vi "rejectAck.vi"(8 "error in (no error)":errorcluster, 10 "InternalCommandId":refnum<class "InternalCommandId.lvclass">, 11 "ElectrometerController in":refnum<class "ElectrometerController.lvclass">) -> (0 "error out":errorcluster, 3 "ElectrometerController out":refnum<class "ElectrometerController.lvclass">)   [LabVIEW 2016, in "ElectrometerController.lvclass"]
uses:
  ElectrometerController.lvclass
  InternalCommandId/InternalCommandId.lvclass
  ts_electrometeruserevents/Typedefs/CommandValue.ctl
  ElectrometerController.lvclass/ElectrometerController.ctl
  ts_electrometeruserevents/PubSubDataEvent/PubSubDataEvent.lvclass
  ts_electrometeruserevents/Typedefs/ElectrometerTypedefs.lvlib
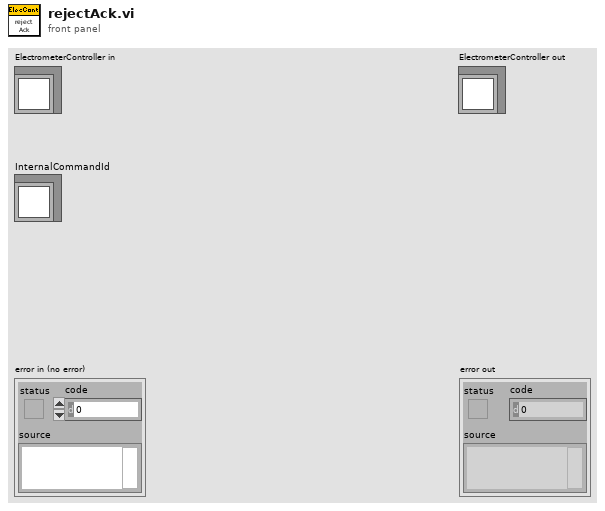
[diagram p1: front panel]
types:
  T1 = typedef "ElectrometerTypedefs.lvlib/CommandValue.ctl" = enum16{"N/A", "Disable", "Enable", "Exit", "GoToStandby", "OnHeartbeat", "OnIncomingMessagingError", "OnInterrupt", "Start", "SetDigitalFilter", "StartScan", "StartScanDt", "StartScanReachIntensity", "StopScan", "SetIntegrationTime", "PerformZeroCalib", "SetRange", "SetMode", "Power"}
  T2 = cluster{"error":i32, "result":string, "ack":i32, "cmdSeqNum":i32, "CommandValue":T1}
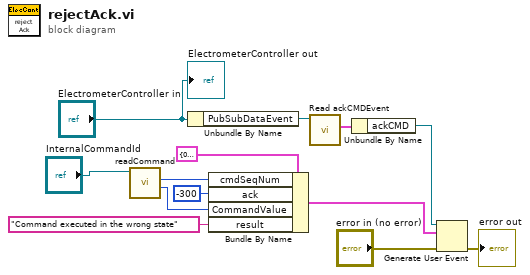
[diagram p0: block diagram]
diagram:
  n1 = call "readCommand.vi"("InternalCommandId in"="InternalCommandId") -> ("CommandValue"=w6:T1, "CommandID"=w4:i32)  [unwired: 7 in, 2 out]
  n2 = Unbundle By Name("ElectrometerController in") -> ("PubSubDataEvent"=w12:refnum<class "PubSubDataEvent.lvclass">)
  n3 = Bundle By Name(cluster=T2 {"error"=0, "result"="", "ack"=0, "cmdSeqNum"=0, "CommandValue"=enum."N/A"} ("event data"), "cmdSeqNum"=w4, "ack"=-300, "CommandValue"=w6, "result"="Command executed in the wrong state") -> (w1:T2)
  n4 = call-dynamic "Read ackCMDEvent.vi"("PubSubDataEvent in"=w12) -> ("ackCMDEvent"=w11:cluster{"ackCMD":refnum<user-event>})  [unwired: 8 in, 2 out]
  n5 = Unbundle By Name(w11) -> ("ackCMD"=w10:refnum<user-event>)
  n6 = Generate User Event(user event=w10, event data cluster=w1, error in="error in (no error)") -> (error out=→"error out":errorcluster)  [unwired: 1 in, 1 out]
  "ElectrometerController out" <- "ElectrometerController in"
